vi "Ver_PN.vi"(0 "aDATA":u8[](array[numeric]) format="%.0x") -> (1 "SubAddress":u8, 2 "Address":u8, 3 "SW ver":string)   [LabVIEW 2017]
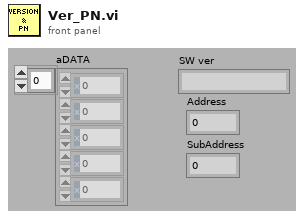
[diagram p1: front panel]
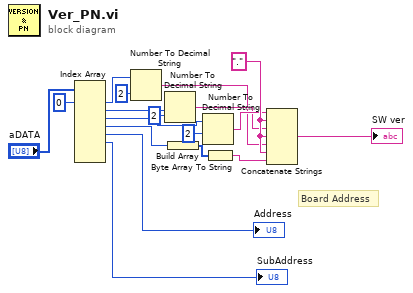
[diagram p0: block diagram]
diagram:
  w13 = "."
  # "Board Address"
  n1 = Index Array(array="aDATA", index #1=0 ("index")) -> (element #1=w16:u8, element #2=w14:u8, element #3=w7:u8, element #4=w12:u8, element #5=→"Address":u8, element #6=→"SubAddress":u8)  [unwired: 7 in, 2 out]
  n2 = Number To Decimal String(number=w16, width (-)=i16 2) -> (decimal integer string=w3:string)
  n3 = Number To Decimal String(number=w14, width (-)=i16 2) -> (decimal integer string=w4:string)
  n4 = Build Array(w12) -> (w11:u8[])
  n5 = Number To Decimal String(number=w7, width (-)=i16 2) -> (decimal integer string=w5:string)
  n6 = Byte Array To String(unsigned byte array=w11) -> (string=w10:string)
  n7 = Concatenate Strings(w5, w13, w4, w13, w3, w13, w10) -> (→"SW ver":string)
